vi "getSPIAccelerometerData.vi"(0 "error in (no error)":errorcluster) -> (1 "X axis":u16, 2 "Y axis":u16, 3 "Z axis":u16, 4 "error out":errorcluster)   [LabVIEW 2012]
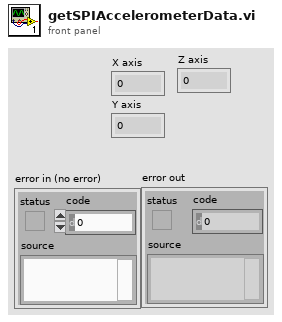
[diagram p1: front panel]
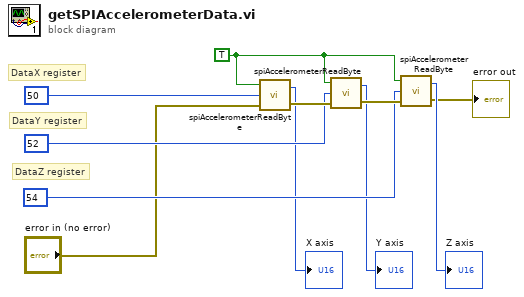
[diagram p0: block diagram]
diagram:
  w9 = TRUE ("Multiple bytes")
  # "DataZ register"
  # "DataY register"
  # "DataX register"
  n1 = call "spiAccelerometerReadByte.vi"("error in (no error)"="error in (no error)", "Address"=50, "Multiple bytes"=w9) -> ("error out"=w11:errorcluster, "Data"=→"X axis":u16)
  n2 = call "spiAccelerometerReadByte.vi"("error in (no error)"=w11, "Address"=52, "Multiple bytes"=w9) -> ("error out"=w10:errorcluster, "Data"=→"Y axis":u16)
  n3 = call "spiAccelerometerReadByte.vi"("error in (no error)"=w10, "Address"=54, "Multiple bytes"=w9) -> ("error out"=→"error out":errorcluster, "Data"=→"Z axis":u16)
